vi "Environment.vi"(8 "Error In":errorcluster, 11 "Environment in":T1) -> (0 "Error Out":errorcluster, 3 "Environment out":T1)   [LabVIEW 2018]
panel:
  in  "Save":bool
  in  "Pressure":dbl=21.0 caption="Numeric" format="%.1f"
  in  "Humidity":dbl=21.0 caption="Numeric" format="%.1f"
  in  "Temperature":dbl=21.0 caption="Numeric" format="%.1f"
  # "Enviroment:"
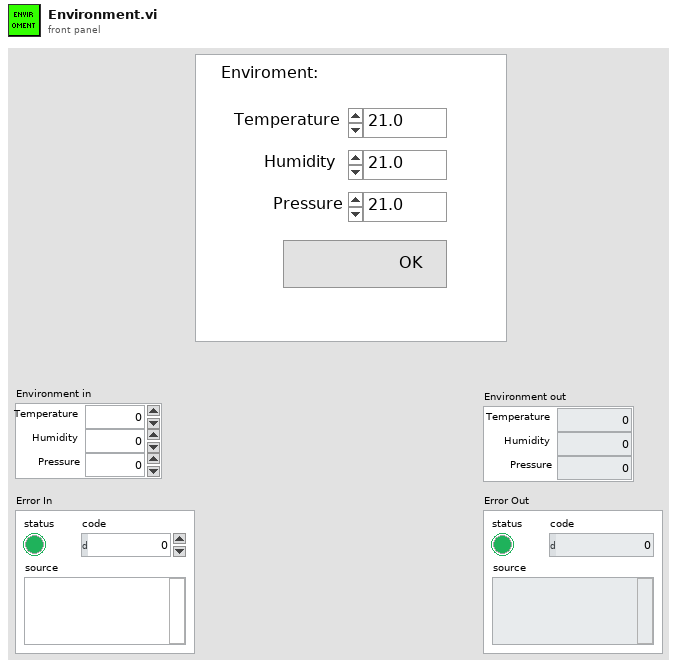
[diagram p1: front panel]
types:
  T1 = cluster{"Temperature":dbl, "Humidity":dbl, "Pressure":dbl}
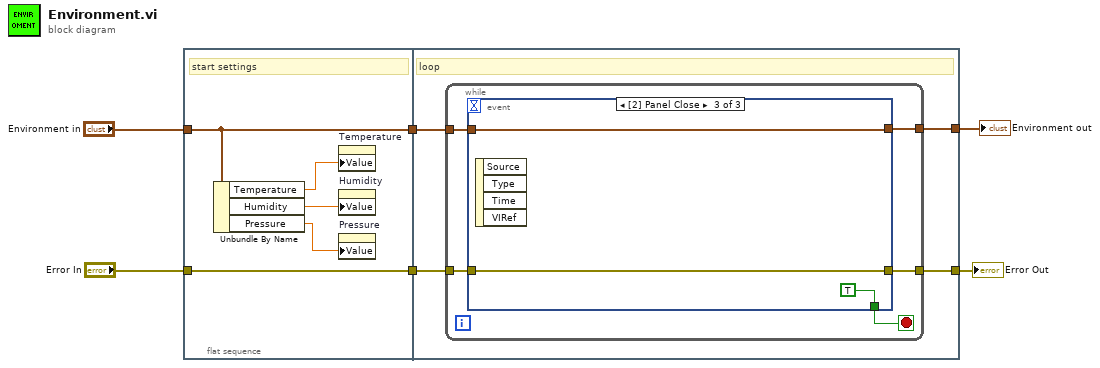
[diagram p0: block diagram]
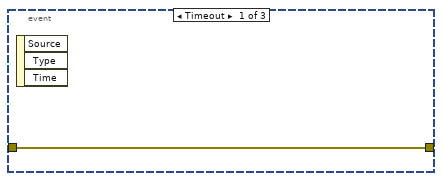
[diagram p2: hidden frame]
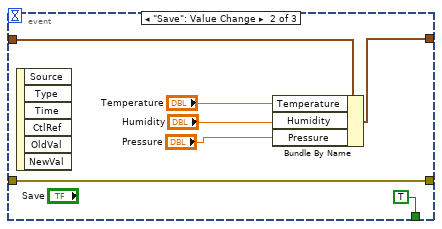
[diagram p3: hidden frame]
diagram:
  n1 = flat-sequence {
    tunnel: [w11] -> w6
    tunnel: "Environment in" -> [w11]
    tunnel: [w7] -> w3
    tunnel: "Error In" -> [w7]
    tunnel: w6 -> [w15]
    tunnel: [w14] -> w4
    tunnel: w3 -> [w12]
    tunnel: [w13] -> w1
    frame #0 {
      # "start settings"
      n2 = Unbundle By Name(w11) -> ("Temperature"=w10:dbl, "Humidity"=w9:dbl, "Pressure"=w8:dbl)
      n3 = property on="Temperature" class="DigNum (strict)"("Value"=w10) -> ()  [unwired: 2 in, 2 out]
      n4 = property on="Humidity" class="DigNum (strict)"("Value"=w9) -> ()  [unwired: 2 in, 2 out]
      n5 = property on="Pressure" class="DigNum (strict)"("Value"=w8) -> ()  [unwired: 2 in, 2 out]
    }
    frame #1 {
      # "loop"
      n6 = while {
        tunnel: w15 -> [w19]
        tunnel: [w18] -> w14
        tunnel: [w17] -> w13
        tunnel: w12 -> [w16]
        stop <- w20 stop-if-true
        n7 = event shown="[2] Panel Close" {
          selector: _ -> [_ _ _]
          dyn-events: _ -> [_ _ _]
          timeout: _ -> [_ _ _]
          tunnel: [_ TRUE TRUE] -> w20
          tunnel: w19 -> [_ w27 w30]
          tunnel: [_ w26 w30] -> w18
          tunnel: [w21 w22 w29] -> w17
          tunnel: w16 -> [w21 w22 w29]
          event Timeout {
            n8 = event-data() -> ()  [unwired: 1 in, 3 out]
          }
          event "Save": Value Change {
            n9 = event-data() -> ()  [unwired: 1 in, 6 out]
            n10 = Bundle By Name(cluster=w27, "Temperature"="Temperature", "Humidity"="Humidity", "Pressure"="Pressure") -> (w26:T1)
          }
          event Panel Close {
            n11 = event-data() -> ()  [unwired: 1 in, 4 out]
          }
        }
      }
    }
  }
  "Environment out" <- w4
  "Error Out" <- w1
